vi "Set Default.vi"(11 "Double in":refnum<class "Double.lvclass">) -> (3 "Double out":refnum<class "Double.lvclass">)   [LabVIEW 2022 SP3, in "Conditum.lvlib" / "Columns.lvlib" / "Double.lvclass"]
uses:
  Double.lvclass
  Double.lvclass/Double.ctl
  Type/Type.lvclass
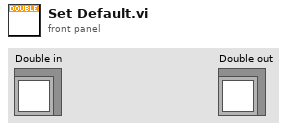
[diagram p1: front panel]
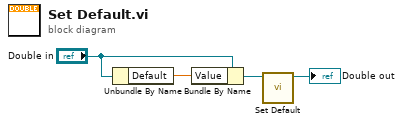
[diagram p0: block diagram]
diagram:
  n1 = Unbundle By Name("Double in") -> ("Default"=w4:dbl)
  n2 = Bundle By Name(cluster="Double in", "Value"=w4) -> (w3:refnum<class "Double.lvclass">)
  n3 = call-parent "Set Default.vi"("Type in"=w3) -> ("Type out"=→"Double out":refnum<class "Double.lvclass">)  [unwired: 10 in]
